vi "example_microFPGA_AnalogIN.vi"() -> ()   [LabVIEW 2021]
panel:
  in  "analog readout channel":u16(ring) items=["channel No 0", "channel No 1", "channel No 2", "channel No 3", "channel No 4", "channel No 5", "channel No 6", "channel No 7"]
  out "analog value read (0 - 65535)":i32=6821
  out "Version":u16=3
  in  "close Application":bool=TRUE
  in  "send parameters":bool
  # "Analog Input value read control"
  # "analog input value read"
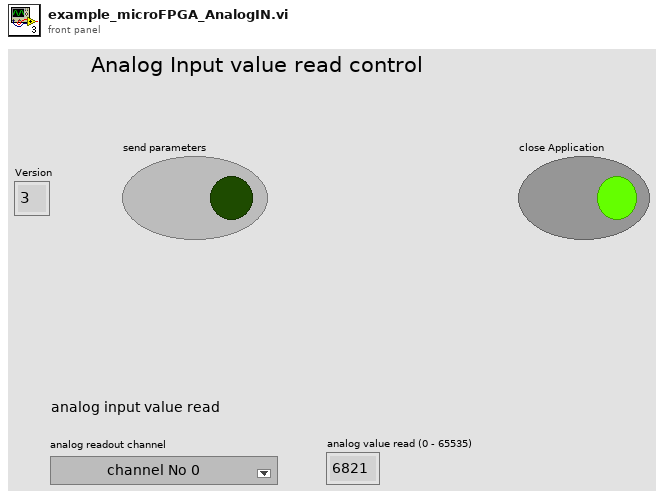
[diagram p1: front panel]
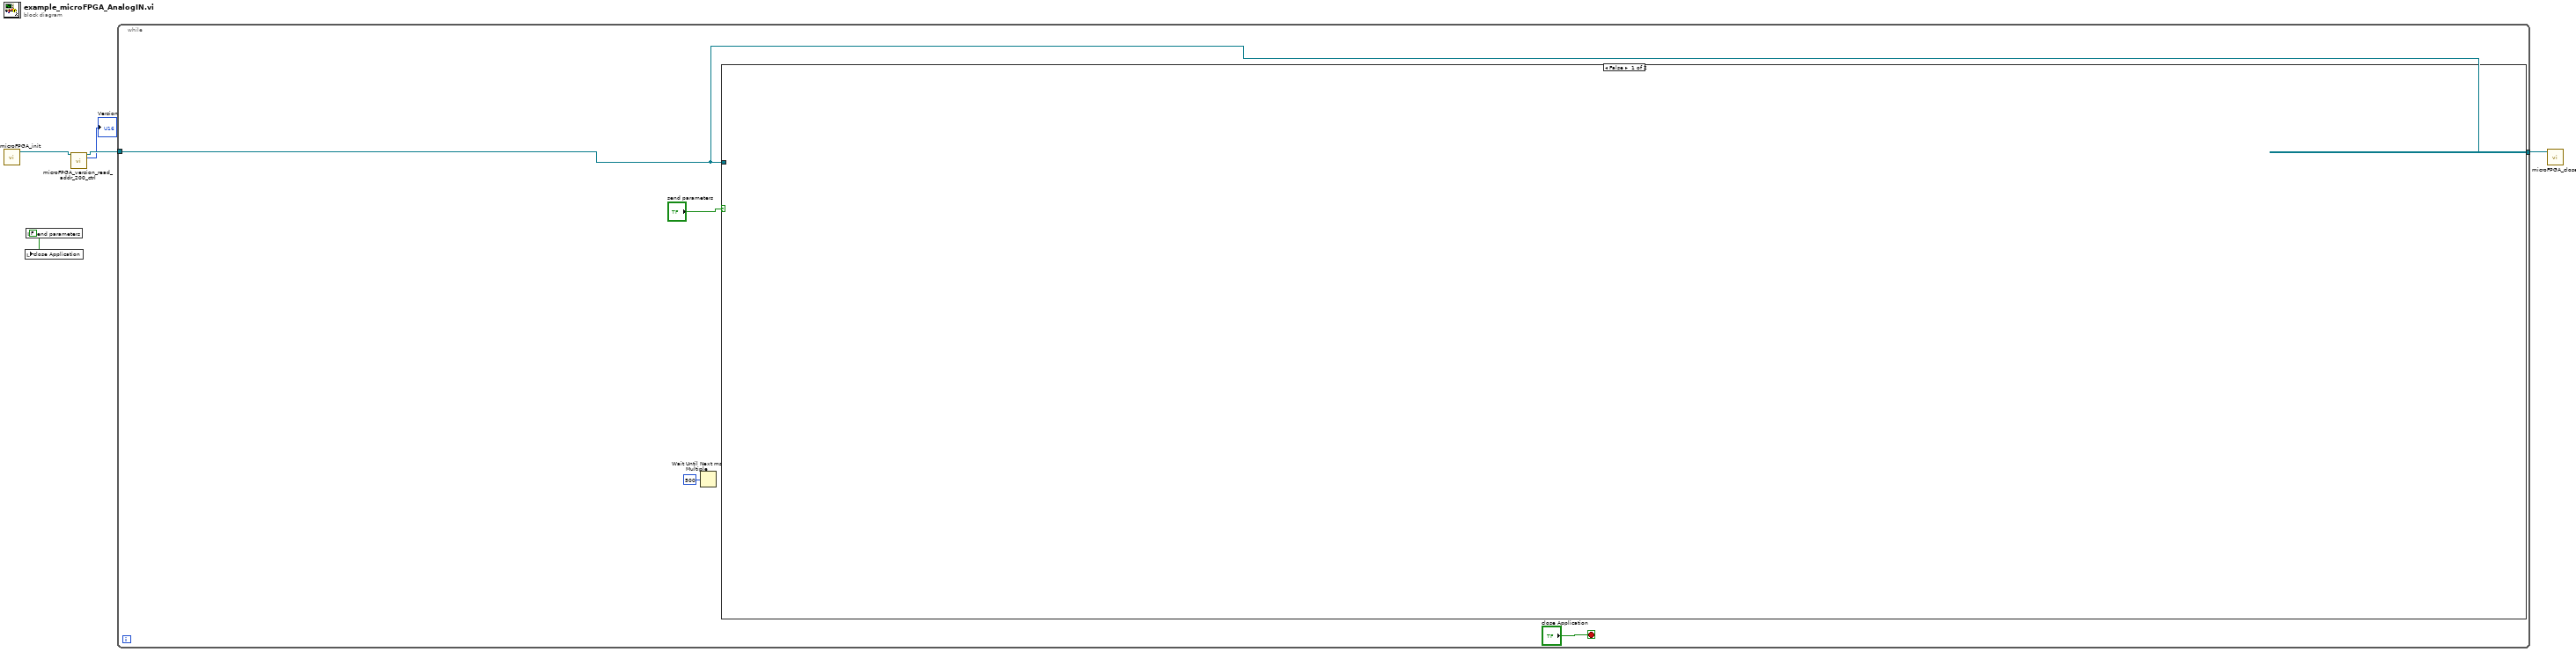
[diagram p0: block diagram]
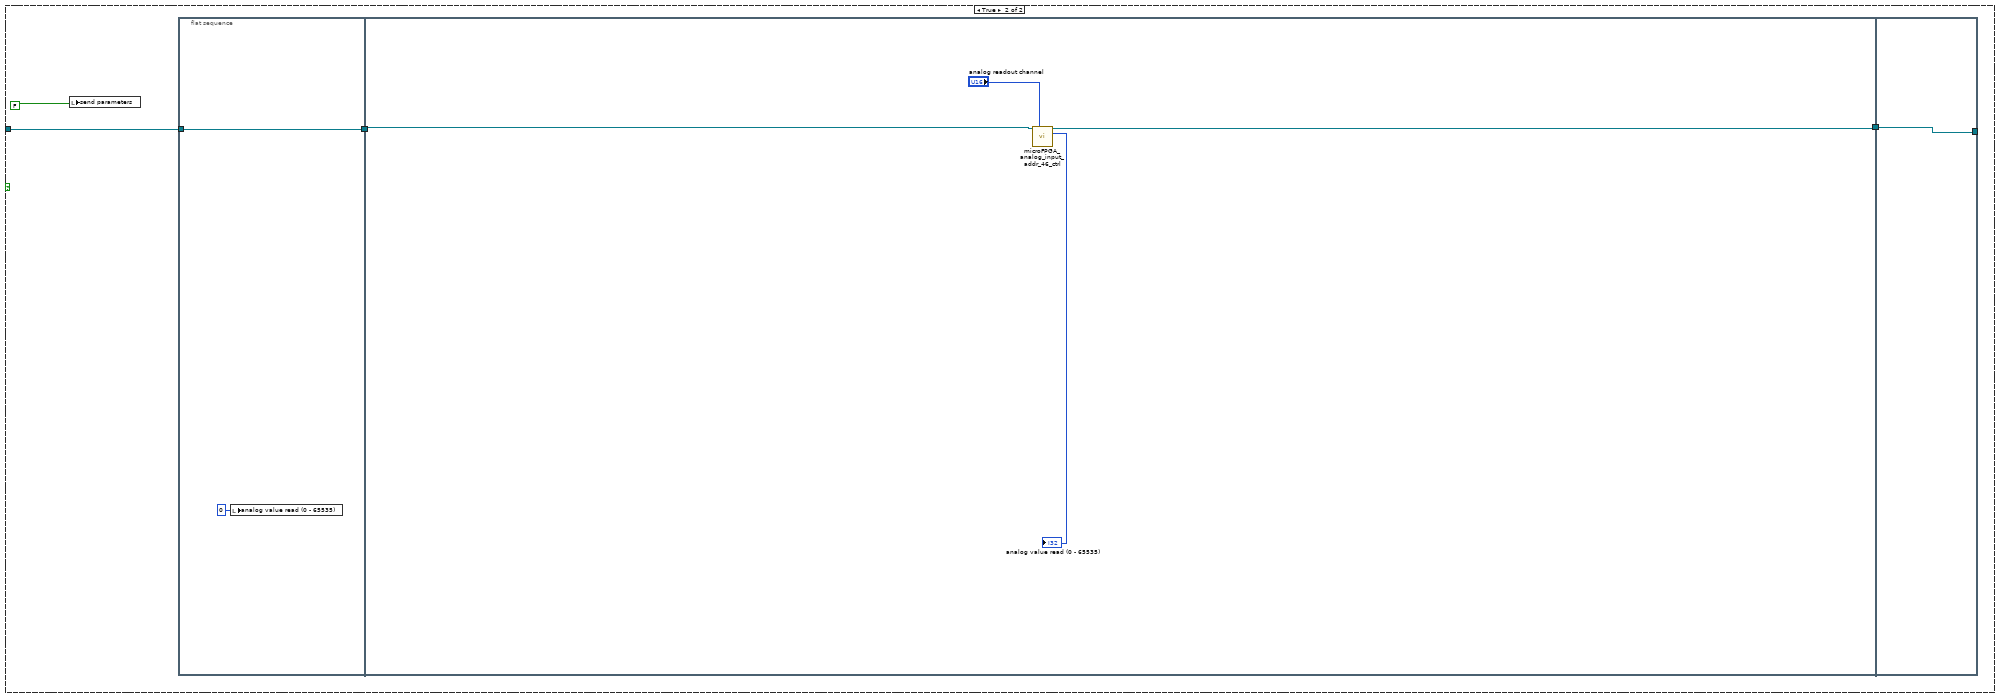
[diagram p2: hidden frame]
diagram:
  w5 = FALSE ("write")
  n1 = call "microFPGA_init.vi"() -> ("VISA resource name out"=w3:refnum<visa-resource-name>)  [unwired: 10 in, 1 out]
  n2 = local write "close Application"(w5) -> ()
  n3 = local write "send parameters"(w5) -> ()
  n4 = call "microFPGA_version_read_addr_200_ctrl.vi"("VISA resource name"=w3) -> ("VISA resource name 2"=w2:refnum<visa-resource-name>, "Version"=→"Version":u16)  [unwired: 12 in, 1 out]
  n5 = while {
    tunnel: w2 -> [w6]
    tunnel: [w6] -> w4
    stop <- "close Application" stop-if-true
    n6 = Wait Until Next ms Multiple(millisecond multiple=u32 500) -> ()  [unwired: 1 out]
    n7 = case shown="False" "send parameters" {
      tunnel: w6 -> [_ w12]
      frame False {
      }
      frame True {
        n8 = local write "send parameters"(FALSE ("write")) -> ()
        n9 = flat-sequence {
          tunnel: w12 -> [w15]
          tunnel: [w15] -> w10
          tunnel: [w17] -> w11
          tunnel: w10 -> [w16]
          tunnel: [w20] -> _
          tunnel: w11 -> [w20]
          frame #0 {
            n10 = local write "analog value read (0 - 65535)"(0 ("analog value read (0 - 65535)")) -> ()
          }
          frame #1 {
            n11 = call "microFPGA_analog_input_addr_46_ctrl.vi"("VISA resource name"=w16, "analog readout channel"="analog readout channel") -> ("VISA resource name 2"=w17:refnum<visa-resource-name>, "analog value read"=→"analog value read (0 - 65535)":i32)  [unwired: 10 in, 2 out]
          }
          frame #2 {
          }
        }
      }
    }
  }
  n12 = call "microFPGA_close.vi"("VISA resource name"=w4) -> ()  [unwired: 11 in]
